vi "Macro Push and Push Tags.vi"(8 "error in (no error)":errorcluster, 11 "Git in":refnum<class "Git.lvclass">) -> (0 "error out":errorcluster, 2 "std out":string, 3 "Git out":refnum<class "Git.lvclass">)   [LabVIEW 2019, in "Git.lvclass"]
uses:
  Git.lvclass
  Git.lvclass/Git.ctl
  <vilib>/Hampel Software Engineering/Git API/Git API/GIT-api.lvclass
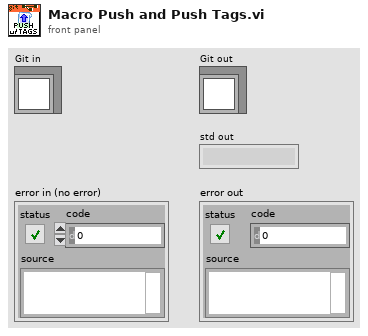
[diagram p1: front panel]
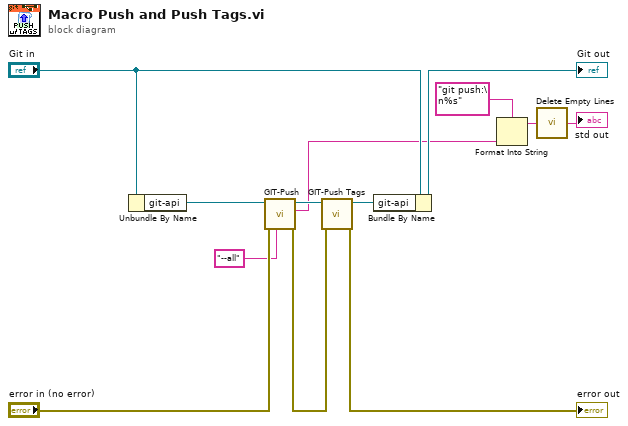
[diagram p0: block diagram]
diagram:
  n1 = Unbundle By Name("Git in") -> ("git-api"=w13:refnum<class "GIT-api.lvclass">)
  n2 = call <vilib>:"GIT-Push.vi"("param"="--all", "error in"="error in (no error)", "Git-API in"=w13) -> ("error out"=w11:errorcluster, "std out"=w3:string, "Git-API out"=w9:refnum<class "GIT-api.lvclass">)  [unwired: 6 in]
  n3 = call <vilib>:"GIT-Push Tags.vi"("error in"=w11, "Git-API in"=w9) -> ("error out"=→"error out":errorcluster, "Git-API out"=w10:refnum<class "GIT-api.lvclass">)  [unwired: 8 in]
  n4 = Bundle By Name(cluster="Git in", "git-api"=w10) -> (→"Git out":refnum<class "Git.lvclass">)
  n5 = Format Into String(format string="git push:\n%s", w3) -> (resulting string=w2:string)  [unwired: 2 in, 1 out]
  n6 = call "Delete Empty Lines.vi"("String"=w2) -> ("delimited string"=→"std out":string)
